vi "StateClimber.vi"(0 "Master State In":T1(ring)) -> ()   [LabVIEW 2020]
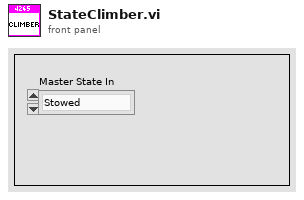
[diagram p1: front panel]
types:
  T1 = enum16{"Stowed", "Balancing", "Scoring", "Hoppering", "Ground", "Shelf"}
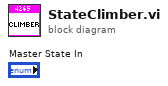
[diagram p0: block diagram]
diagram:
